vi "Drum Red.vi"(0 "ROI Descriptor (Line Profile 1)":T1={"Global Rectangle"=[300, 289, 323, 384], "Contours"=[{"ID"=enum."External", "Type"=2, "Coordinates"=[322, 289, 300, 383]}]} {"Contours"."Type" items=["No Selection", "Point", "Line", "Rectangle", "Oval", "Polygon", "Freehand Region", "Annulus", "Unused2", "Unused3", "Broken Line", "Freehand Line", "Rotated Rectangle"]}, 1 "Color Mode (Line Profile 1)":u16(ring)=3 items=["RGB", "HSL", "HSV", "HSI"], 7 "error in":errorcluster) -> (20 "Line Profile (Line Profile 1)":u8[][](array[numeric]), 27 "error out":errorcluster)   [LabVIEW 2009]
panel:
  out "Image Out":T2(plugin-control)
  out "Line Profile Graph":u8[][](graph) caption="Line Profile"
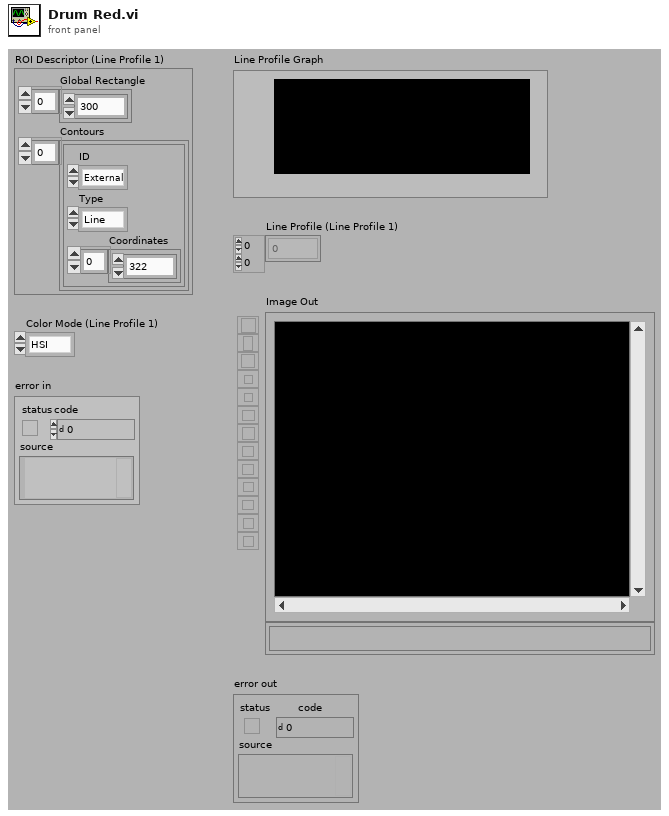
[diagram p1: front panel]
types:
  T1 = cluster{"Global Rectangle":i32[], "Contours":cluster{"ID":enum32{"External", "Internal"}, "Type":u32, "Coordinates":i32[]}[]}
  T2 = typedef "IMAQ Image.ctl" = refnum<image>
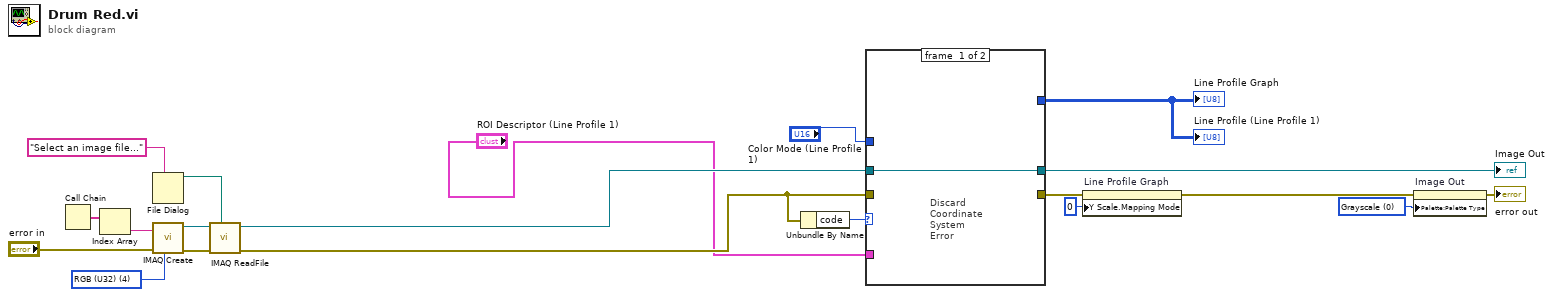
[diagram p0: block diagram]
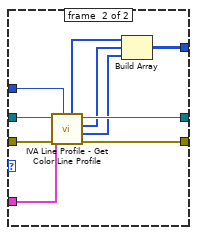
[diagram p2: hidden frame]
diagram:
  w2 = u32 0 items=["Grayscale", "Binary", "Gradient", "Rainbow", "Temperature", "User Defined"] ("Palette")
  w17 = u32 4 items=["Grayscale (U8)", "Grayscale (I16)", "Grayscale (SGL)", "Complex (CSG)", "RGB (U32)", "HSL (U32)", "RGB (U64)"] ("Image Type")
  n1 = Call Chain() -> (call chain=w13:string[])
  n2 = Index Array(array=w13) -> (element=w12:string)  [unwired: 1 in]
  n3 = File Dialog(7:"Select an image file..." ("prompt")) -> (3:w16:path)  [unwired: 1 in, 8 out]
  n4 = call "IMAQ Create"("Image Name"=w12, "Image Type"=w17, "error in (no error)"="error in") -> ("New Image"=w19:T2, "error out"=w18:errorcluster)  [unwired: 1 in, 1 out]
  n5 = call "IMAQ ReadFile"("File Path"=w16, "error in (no error)"=w18, "Image"=w19) -> ("error out"=w20:errorcluster, "Image Out"=w7:T2)  [unwired: 2 in, 5 out]
  n6 = Unbundle By Name(w20) -> ("code"=w4:i32)
  n7 = case shown="Default" w4 {
    tunnel: w20 -> [_ w31]
    tunnel: [_ w30] -> w10
    tunnel: "Color Mode (Line Profile 1)" -> [_ w29]
    tunnel: [w21 w28] -> w3
    tunnel: w7 -> [w21 w27]
    tunnel: [_ w23] -> w6
    tunnel: "ROI Descriptor (Line Profile 1)" -> [_ w22]
    frame #0 {
      # "Discard\nCoordinate\nSystem\nError"
    }
    frame #1 {
      n8 = call <vilib>:"IVA Line Profile - Get Color Line Profile.vi"("Color Mode"=w29, "error in (no error)"=w31, "ROI Descriptor"=w22, "Image In"=w27) -> ("error out"=w30:errorcluster, "Blue or Luma Pixels"=w24:u8[], "Green or Sat Pixels"=w25:u8[], "Image Out"=w28:T2, "Red or Hue Pixels"=w26:u8[])  [unwired: 3 out]
      n9 = Build Array(w26, w25, w24) -> (w23:u8[][])
    }
  }
  "Line Profile Graph" <- w6
  "Line Profile (Line Profile 1)" <- w6
  "Image Out" <- w3
  n10 = property on="Line Profile Graph"(error in=w10, "Y Scale.Mapping Mode"=u8 0) -> (error out=w9:errorcluster)  [unwired: 1 in, 1 out]
  n11 = property on="Image Out" class="ImageControl"(error in=w9, "Palette:Palette Type"=w2) -> (error out=→"error out":errorcluster)  [unwired: 1 in, 1 out]
